vi "getCluster.vi"(0 "数据":string[][](array[string]), 5 "检定次数":i32=1, 9 "压力点个数":i32, 11 "传感器索引（1开始）":i32=1, 12 "R5-1":dbl, 14 "理论 K":dbl) -> (1 "迟滞mV":dbl[](array[numeric]), 2 "线性误差":dbl[](array[numeric]), 3 "截距数组":dbl[](array[numeric]), 4 "结果簇":cluster{dbl[], dbl[]}[](array[cluster]), 6 "曲线信息":string[](array[string]), 10 "Rx":dbl[](array[numeric]), 13 "系统误差mV":dbl[](array[numeric]), 15 "斜率数组":dbl[](array[numeric]))   [LabVIEW 2017]
uses:
  348cd42a-b631-4f36-b7c5-add1cd6ca5ad.vi
  <vilib>/Array/Sort 2D Array - Pop Stack.vi
  <vilib>/Array/Sort 2D Array - Push Stack.vi
panel:
  out "数组":dbl[][](array[numeric])
  in  "反tmp":dbl[][](array[numeric])
  in  "正tmp":dbl[][](array[numeric])
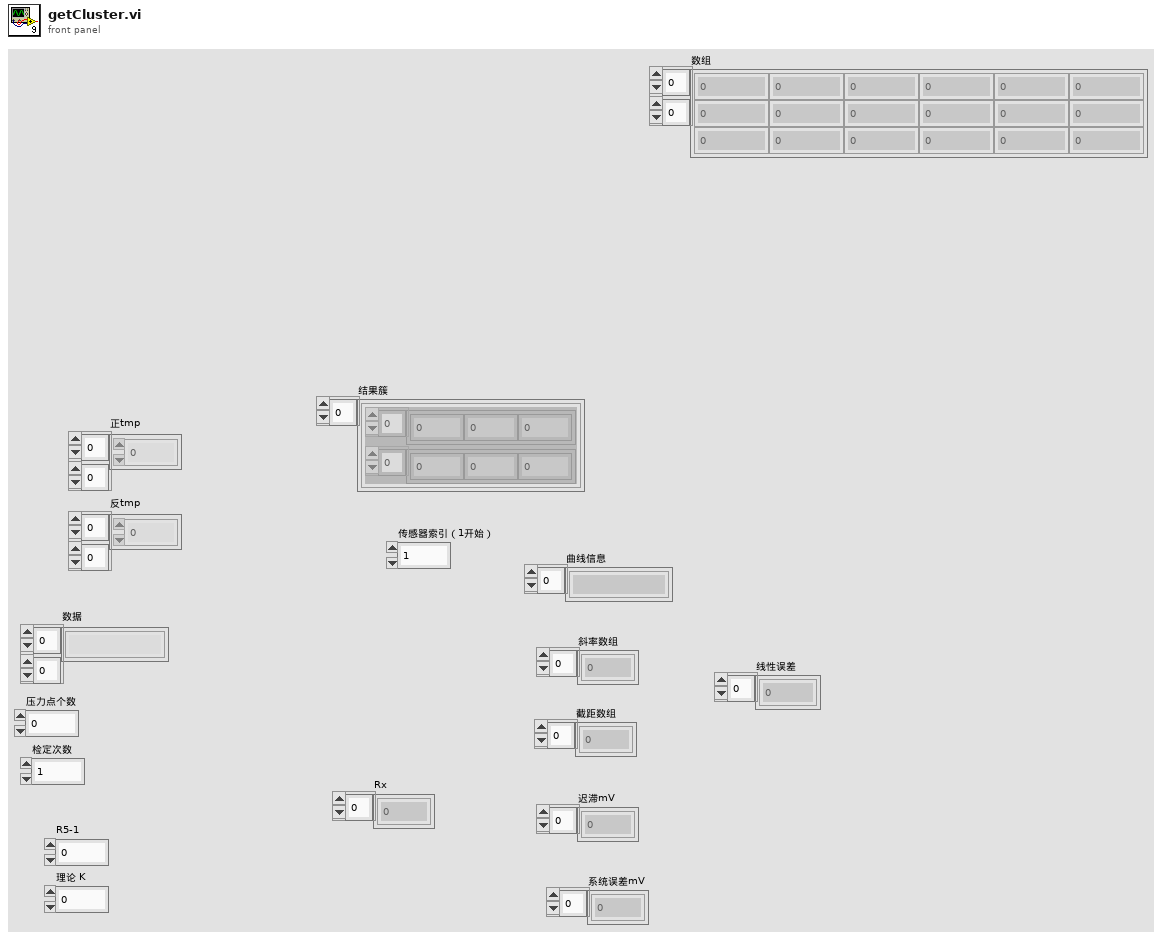
[diagram p1: front panel]
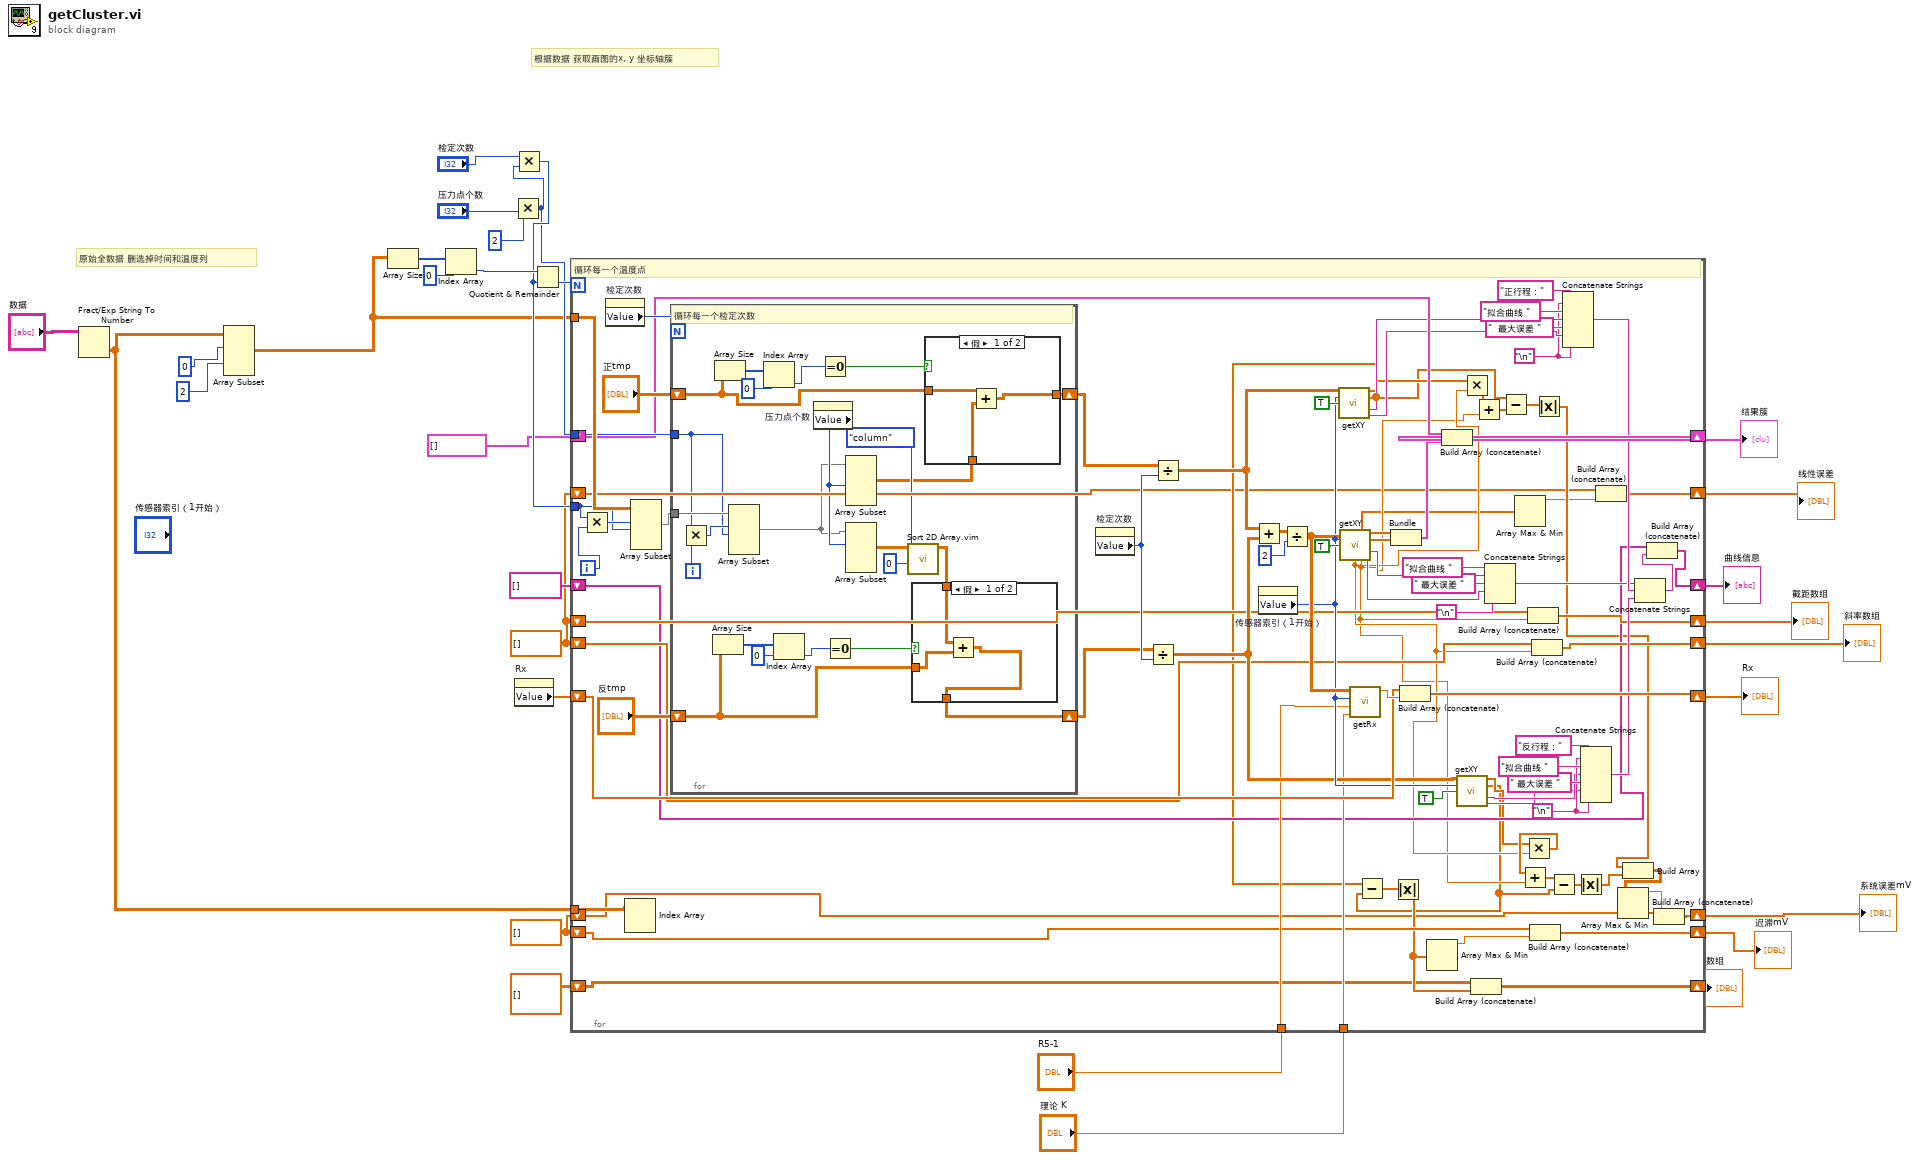
[diagram p0: block diagram]
diagram:
  w4 = dbl[] []
  w2 = dbl[] []
  # "原始全数据 删选掉时间和温度列"
  # "根据数据 获取画图的x, y 坐标轴簇"
  n1 = Fract/Exp String To Number(string="数据") -> (number=w8:dbl[][])  [unwired: 3 in, 1 out]
  n2 = Array Subset(array=w8, index (row)=0 ("长度"), index (col)=2 ("索引")) -> (w18:dbl[][])  [unwired: 2 in]
  n3 = Array Size(array=w18) -> (size(s)=w26:i32[])
  n4 = Index Array(array=w26, index=0 ("索引")) -> (element=w24:i32)
  n5 = Multiply(x=2, y="压力点个数") -> (x*y=w21:i32)
  n6 = Multiply(x="检定次数", y=w21) -> (x*y=w22:i32)
  n7 = property on="Rx" class="Arr (严格)"() -> ("Value"=w15:dbl[])  [unwired: 2 in, 2 out]
  n8 = Quotient & Remainder(x=w24, y=w22) -> (floor(x/y)=w27:i32)  [unwired: 1 out]
  n9 = for "循环每一个温度点" {
    N: w27 -> [_]
    tunnel: w18 -> [w119]
    tunnel: w22 -> [w116]
    tunnel: w21 -> [w113]
    shift-right: [w106] -> w19
    shift-left: cluster{dbl[], dbl[]}[] [] -> [w111]
    shift-right: [w62] -> w10
    shift-left: string[] [] -> [w64]
    shift-right: [w94] -> w16
    shift-left: w15 -> [w95]
    shift-right: [w69] -> w14
    shift-left: w2 -> [w70]
    tunnel: "理论 K" -> [w68]
    tunnel: "R5-1" -> [w67]
    shift-right: [w65] -> w11
    shift-left: w2 -> [w66]
    tunnel: w8 -> [w61]
    shift-right: [w59] -> w7
    shift-left: w4 -> [w58]
    shift-right: [w55] -> w5
    shift-left: dbl[][] [] -> [w54]
    shift-right: [w37] -> w3
    shift-left: w4 -> [w36]
    shift-right: [w33] -> w1
    shift-left: w2 -> [w32]
    i -> [w118]
    w81 = "\n"
    w87 = "\n"
    # "循环每一个温度点"
    n10 = Multiply(x=w116, y=w118) -> (x*y=w117:i32)
    n11 = property on="检定次数" class="DigNum (严格)"() -> ("Value"=w115:i32)  [unwired: 2 in, 2 out]
    n12 = Index Array(array=w61) -> ()  [unwired: 2 in, 1 out]
    n13 = Array Subset(array=w119, index (row)=w117, length (row)=w116) -> (w114:dbl[][])  [unwired: 2 in]
    n14 = for {
      N: w115 -> [_]
      tunnel: w114 -> [w138]
      tunnel: w113 -> [w135]
      shift-right: [w129] -> w74
      shift-left: "正tmp" -> [w128]
      shift-right: [w121] -> w73
      shift-left: "反tmp" -> [w120]
      i -> [w137]
      # "循环每一个检定次数"
      n15 = Multiply(x=w135, y=w137) -> (x*y=w136:i32)
      n16 = Array Size(array=w120) -> (size(s)=w127:i32[])
      n17 = Array Size(array=w128) -> (size(s)=w133:i32[])
      n18 = Array Subset(array=w138, index (row)=w136, length (row)=w135) -> (w134:dbl[][])  [unwired: 2 in]
      n19 = Index Array(array=w133, index=0 ("索引")) -> (element=w131:i32)
      n20 = Index Array(array=w127, index=0 ("索引")) -> (element=w125:i32)
      n21 = property on="压力点个数" class="DigNum (严格)"() -> ("Value"=w142:i32)  [unwired: 2 in, 2 out]
      n22 = Equal To 0?(x=w131) -> (x = 0?=w130:bool)
      n23 = Equal To 0?(x=w125) -> (x = 0?=w124:bool)
      n24 = Array Subset(array=w134, length (row)=w142) -> (w123:dbl[][])  [unwired: 3 in]
      n25 = Array Subset(array=w134, index (row)=w142) -> (w139:dbl[][])  [unwired: 3 in]
      n26 = call "Sort 2D Array.vim"("index"=0, "dimension to index (column)"=enum16{"column", "row"}."column", "2D array"=w139) -> ("sorted 2D array"=w122:dbl[][])  [unwired: 7 in, 1 out]
      n27 = case shown="假" w124 {
        tunnel: w122 -> [w144 w146]
        tunnel: [w143 w146] -> w121
        tunnel: w120 -> [w145 _]
        frame False {
          n28 = Add(x=w144, y=w145) -> (x+y=w143:dbl[][])
        }
        frame True {
        }
      }
      n29 = case shown="假" w130 {
        tunnel: w123 -> [w149 w150]
        tunnel: [w147 w150] -> w129
        tunnel: w128 -> [w148 _]
        frame False {
          n30 = Add(x=w148, y=w149) -> (x+y=w147:dbl[][])
        }
        frame True {
        }
      }
    }
    n31 = property on="检定次数" class="DigNum (严格)"() -> ("Value"=w75:i32)  [unwired: 2 in, 2 out]
    n32 = Divide(x=w73, y=w75) -> (x/y=w72:dbl[][])
    n33 = Divide(x=w74, y=w75) -> (x/y=w71:dbl[][])
    n34 = Add(x=w71, y=w72) -> (x+y=w109:dbl[][])
    n35 = property on="传感器索引（1开始）" class="DigNum (严格)"() -> ("Value"=w86:i32)  [unwired: 2 in, 2 out]
    n36 = Divide(x=w109, y=2) -> (x/y=w97:dbl[][])
    n37 = call "getXY.vi"("数据"=w71, "传感器索引"=w86, "是否需要计算拟合曲线"=TRUE) -> ("x"=w52:dbl[], "y"=w50:dbl[], "拟合曲线"=w90:string, "最大误差率"=w89:string)  [unwired: 5 in, 4 out]
    n38 = call "getXY.vi"("数据"=w97, "传感器索引"=w86, "是否需要计算拟合曲线"=TRUE) -> ("绝对偏差（mV）"=w35:dbl[], "x"=w104:dbl[], "y"=w103:dbl[], "拟合曲线"=w102:string, "slope"=w46:dbl, "intercept"=w45:dbl, "最大误差率"=w99:string)  [unwired: 5 in, 1 out]
    n39 = call "getRx.vi"("理论 K"=w68, "R5-1"=w67, "传感器索引"=w86, "数据"=w97) -> ("Rx"=w96:dbl)  [unwired: 7 in]
    n40 = Bundle("x"=w104, "y"=w103) -> (w107:cluster{"x":dbl[], "y":dbl[]})  [unwired: 1 in]
    n41 = Build Array (concatenate)(w95, w96) -> (w94:dbl[])
    n42 = Build Array (concatenate)(w111, w107) -> (w106:cluster{"x":dbl[], "y":dbl[]}[])
    n43 = call "getXY.vi"("数据"=w72, "传感器索引"=w86, "是否需要计算拟合曲线"=TRUE) -> ("x"=w47:dbl[], "y"=w43:dbl[], "拟合曲线"=w80:string, "最大误差率"=w79:string)  [unwired: 5 in, 4 out]
    n44 = Subtract(x=w50, y=w43) -> (x-y=w60:dbl[])
    n45 = Absolute Value(x=w60) -> (abs(x)=w56:dbl[])
    n46 = Array Max & Min(array=w56) -> (max value=w57:dbl)  [unwired: 3 out]
    n47 = Multiply(x=w52, y=w46) -> (x*y=w53:dbl[])
    n48 = Build Array (concatenate)(w54, w56) -> (w55:dbl[][])
    n49 = Add(x=w53, y=w45) -> (x+y=w51:dbl[])
    n50 = Concatenate Strings("拟合曲线 " ("字符串"), w102, " 最大误差 " ("字符串"), w99, "\n") -> (w76:string)
    n51 = Subtract(x=w50, y=w51) -> (x-y=w49:dbl[])
    n52 = Array Max & Min(array=w35) -> (max value=w34:dbl)  [unwired: 3 out]
    n53 = Multiply(x=w47, y=w46) -> (x*y=w48:dbl[])
    n54 = Add(x=w48, y=w45) -> (x+y=w44:dbl[])
    n55 = Build Array (concatenate)(w66, w45) -> (w65:dbl[])
    n56 = Build Array (concatenate)(w58, w57) -> (w59:dbl[])
    n57 = Build Array (concatenate)(w70, w46) -> (w69:dbl[])
    n58 = Absolute Value(x=w49) -> (abs(x)=w40:dbl[])
    n59 = Subtract(x=w44, y=w43) -> (x-y=w42:dbl[])
    n60 = Concatenate Strings("正行程：" ("字符串"), w87, "拟合曲线 " ("字符串"), w90, "  最大误差 " ("字符串"), w89, w87) -> (w77:string)
    n61 = Absolute Value(x=w42) -> (abs(x)=w41:dbl[])
    n62 = Concatenate Strings("反行程：" ("字符串"), w81, "拟合曲线 " ("字符串"), w80, " 最大误差 " ("字符串"), w79, w81) -> (w78:string)
    n63 = Build Array (concatenate)(w32, w34) -> (w33:dbl[])
    n64 = Build Array(w40, w41) -> (w39:dbl[][])
    n65 = Array Max & Min(array=w39) -> (max value=w38:dbl)  [unwired: 3 out]
    n66 = Concatenate Strings(w76, w77, w78) -> (w63:string)
    n67 = Build Array (concatenate)(w64, w63) -> (w62:string[])
    n68 = Build Array (concatenate)(w36, w38) -> (w37:dbl[])
  }
  "结果簇" <- w19
  "Rx" <- w16
  "斜率数组" <- w14
  "截距数组" <- w11
  "曲线信息" <- w10
  "迟滞mV" <- w7
  "数组" <- w5
  "系统误差mV" <- w3
  "线性误差" <- w1
